vi "Limit Value.vi"(0 "Value":dbl, 1 "Limit":dbl) -> (6 "Limited Value":dbl)   [LabVIEW 2020]
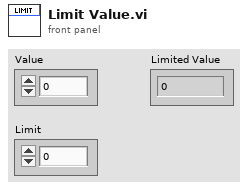
[diagram p1: front panel]
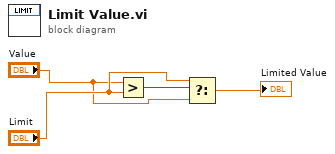
[diagram p0: block diagram]
diagram:
  n1 = Greater?(x="Value", y="Limit") -> (0:w4:bool)
  n2 = Select(t="Limit", s=w4, f="Value") -> (s? t:f=→"Limited Value":dbl)
